vi "Seconds Breakdown.vi"(11 "Total Time in Seconds":dbl) -> (0 "Message":string, 1 "Seconds":dbl, 2 "Minutes":dbl, 3 "Hours":dbl, 5 "Warning":bool)   [LabVIEW 2012]
panel:
  # "Converts seconds into separate indicators of hours, minutes, and seconds.  \nAlerts users with LED and message if time exceeds 1 hour."
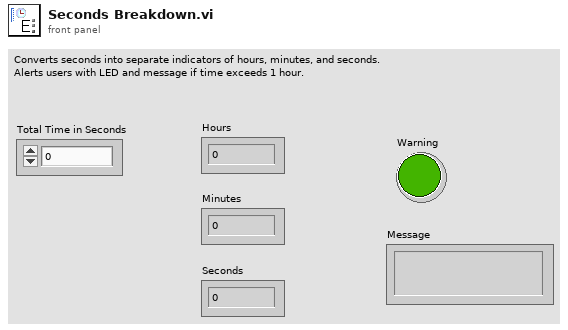
[diagram p1: front panel]
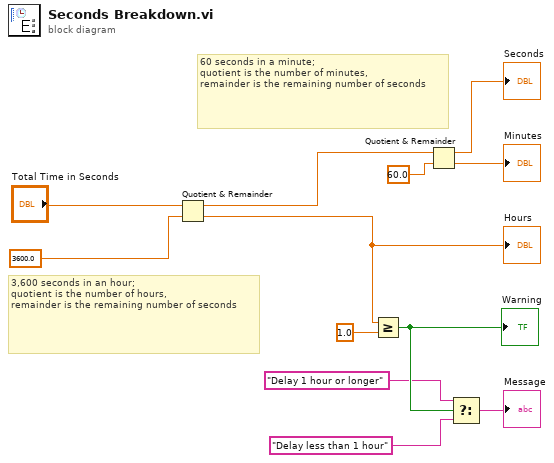
[diagram p0: block diagram]
diagram:
  # "60 seconds in a minute;\nquotient is the number of minutes,\nremainder is the remaining number of seconds"
  # "3,600 seconds in an hour;\nquotient is the number of hours,\nremainder is the remaining number of seconds"
  n1 = Quotient & Remainder(x="Total Time in Seconds", y=3600.0) -> (x-y*floor(x/y)=w11:dbl, floor(x/y)=w6:dbl)
  "Hours" <- w6
  n2 = Greater Or Equal?(x=w6, y=1.0) -> (x >= y?=w4:bool)
  "Warning" <- w4
  n3 = Quotient & Remainder(x=w11, y=60.0) -> (x-y*floor(x/y)=→"Seconds":dbl, floor(x/y)=→"Minutes":dbl)
  n4 = Select(t="Delay 1 hour or longer", s=w4, f="Delay less than 1 hour") -> (s? t:f=→"Message":string)
